vi "Set_Wavelength.vi"(8 "error in (no error)":errorcluster, 10 "Wavelength (m)":dbl, 11 "Thorlabs_PM100D in":refnum<class "Thorlabs_PM100D.lvclass">) -> (0 "error out":errorcluster, 3 "Thorlabs_PM100D out":refnum<class "Thorlabs_PM100D.lvclass">)   [LabVIEW 2020, in "Thorlabs_PM100D.lvclass"]
uses:
  <instrlib>/Classes/Powermeter/Thorlabs_PM100D/Thorlabs_PM100D.lvclass
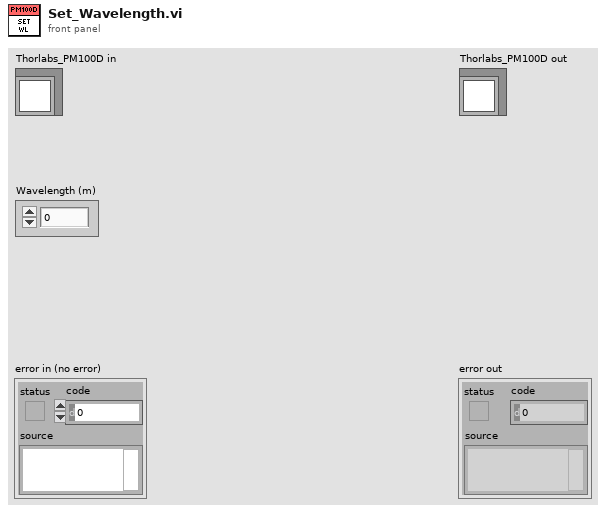
[diagram p1: front panel]
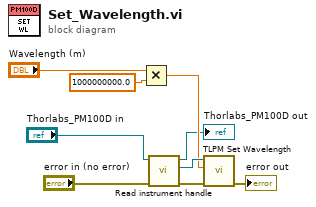
[diagram p0: block diagram]
diagram:
  n1 = Multiply(x="Wavelength (m)", y=1000000000.0) -> (x*y=w5:dbl)
  n2 = call-dynamic "Read instrument handle.vi"("error in (no error)"="error in (no error)", "Thorlabs_PM100D in"="Thorlabs_PM100D in") -> ("error out"=w4:errorcluster, "instrument handle"=w8:refnum<visa-resource-name>, "Thorlabs_PM100D out"=→"Thorlabs_PM100D out":refnum<class "Thorlabs_PM100D.lvclass">)  [unwired: 7 in]
  n3 = call <instrlib>:"TLPM Set Wavelength.vi"("error in (no error)"=w4, "Wavelength (0.0)"=w5, "instrument handle"=w8) -> ("error out"=→"error out":errorcluster)  [unwired: 7 in, 1 out]
